vi "Intake Teleop.vi"(10 "Button Presses":bool[](array[boolean]), 11 "Axes":dbl[](array[numeric])) -> ()   [LabVIEW 2019]
uses:
  Pivot Position.ctl
panel:
  in  "Pivot Starting Pos":T1
  in  "Setpoint":dbl
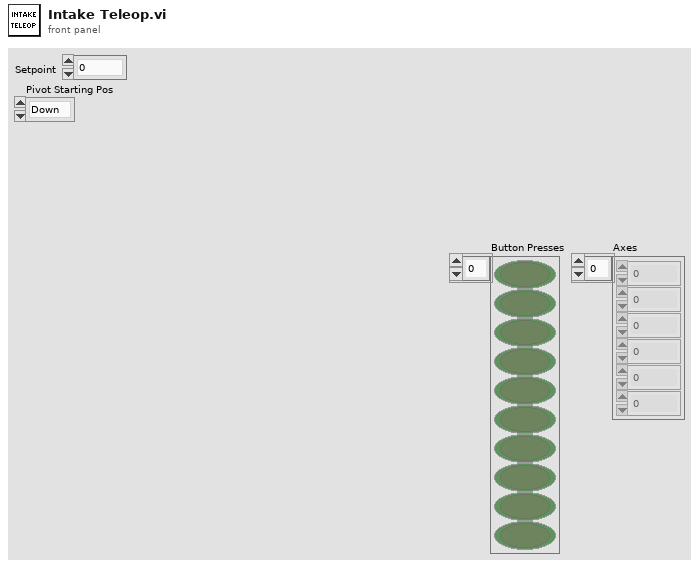
[diagram p1: front panel]
types:
  T1 = typedef "Pivot Position.ctl" = enum16{"Down", "Up"}
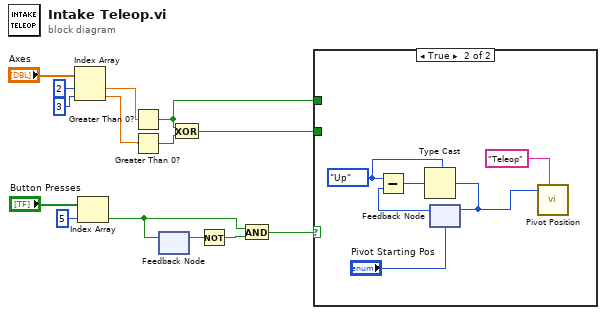
[diagram p0: block diagram]
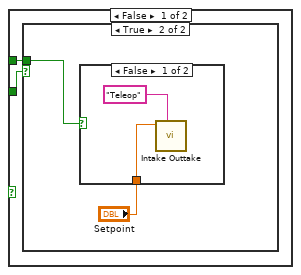
[diagram p2: hidden frame]
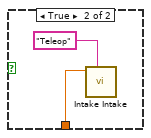
[diagram p4: hidden frame]
diagram:
  n1 = Index Array(array="Axes", index #1=2 ("index"), index #2=3 ("index")) -> (element #1=w4:dbl, element #2=w5:dbl)
  n2 = Index Array(array="Button Presses", index=5) -> (element=w7:bool)
  n3 = Greater Than 0?(x=w4) -> (x > 0?=w1:bool)
  n4 = Greater Than 0?(x=w5) -> (x > 0?=w3:bool)
  n5 = feedback-in #1(w7) -> ()
  n6 = feedback #1() -> (w9:bool)  [unwired: 1 in]
  n7 = Exclusive Or(1:w3, 2:w1) -> (0:w2:bool)
  n8 = Not(x=w9) -> (.not. x?=w8:bool)
  n9 = And(x=w7, y=w8) -> (x .and. y?=w6:bool)
  n10 = case shown="True" w6 {
    tunnel: w2 -> [w16 _]
    tunnel: w1 -> [w15 _]
    frame False {
      n11 = case shown="True" w16 {
        tunnel: w15 -> [_ w18]
        frame False {
        }
        frame True {
          n12 = case shown="False" w18 {
            tunnel: "Setpoint" -> [w20 w22]
            frame False {
              n13 = call "Intake Outtake.vi"("Description"="Teleop", "Setpoint"=w20) -> ()  [unwired: 9 in, 1 out]
            }
            frame True {
              n14 = call "Intake Intake.vi"("Description"="Teleop", "Setpoint"=w22) -> ()  [unwired: 9 in, 1 out]
            }
          }
        }
      }
    }
    frame True {
      w24 = Pivot_Position."Up" ("x")
      n15 = feedback #2("Pivot Starting Pos") -> (w27:T1)
      n16 = Subtract(x=w24, y=w27) -> (x-y=w25:u16)
      n17 = Type Cast(type=w24, x=w25) -> (*(type *) &x=w23:T1)
      n18 = feedback-in #2(w23) -> ()
      n19 = call "Pivot Position.vi"("Description"="Teleop", "Pivot Position"=w23) -> ()  [unwired: 9 in, 1 out]
    }
  }
